vi "solar_app Version.vi"() -> (2 "SOLAR Version":string)   [LabVIEW 2018]
doc: "This VI description contains the VI Package version of SOLAR. This is set as a pre build action."
panel:
  in  "vip":string="16.3.3.7"
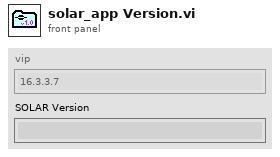
[diagram p1: front panel]
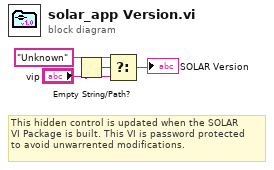
[diagram p0: block diagram]
diagram:
  # "This hidden control is updated when the SOLAR\nVI Package is built. This VI is password protected\nto avoid unwarrented modifications."
  n1 = Empty String/Path?(string/path="vip") -> (empty?=w4:bool)
  n2 = Select(t="Unknown", s=w4, f="vip") -> (s? t:f=→"SOLAR Version":string)
